vi "GetEventForceActuatorForceWarningField.vi"(10 "Event Data":string, 11 "Cluster in":refnum<vi>) -> (3 "Array":string[](array[string]))   [LabVIEW 2016]
uses:
  SALLV_m1m3/DataTypes/logevent_ForceActuatorForceWarning.ctl
  SALLV_m1m3/SALLV_m1m3.lvlib
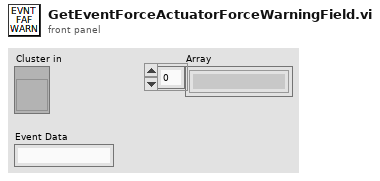
[diagram p1: front panel]
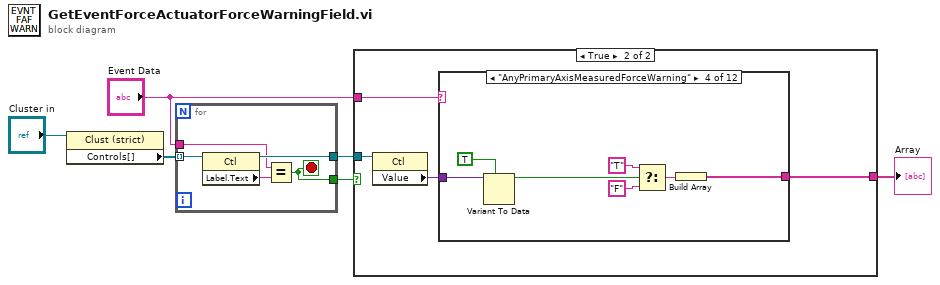
[diagram p0: block diagram]
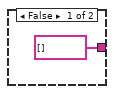
[diagram p2: hidden frame]
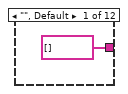
[diagram p3: hidden frame]
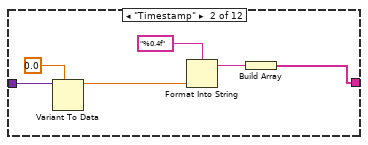
[diagram p4: hidden frame]
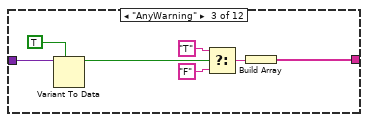
[diagram p5: hidden frame]
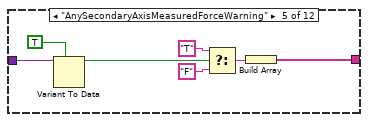
[diagram p6: hidden frame]
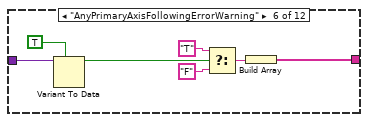
[diagram p7: hidden frame]
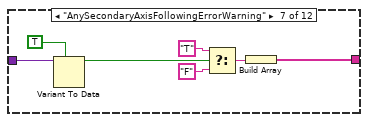
[diagram p8: hidden frame]
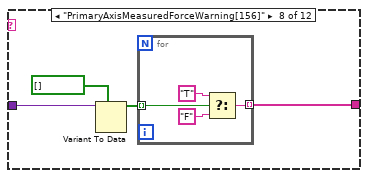
[diagram p9: hidden frame]
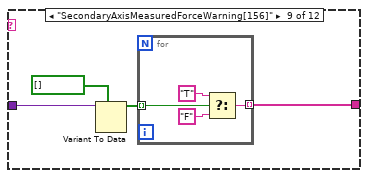
[diagram p10: hidden frame]
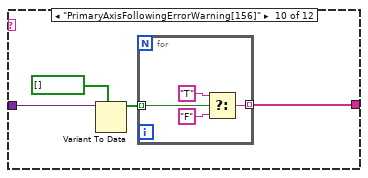
[diagram p11: hidden frame]
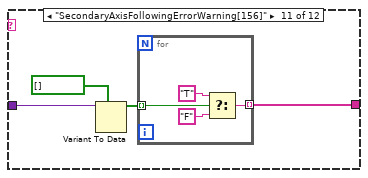
[diagram p12: hidden frame]
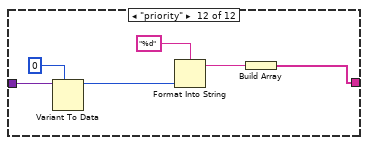
[diagram p13: hidden frame]
diagram:
  n1 = property on="Property Node" class="Clust (strict)"(reference="Cluster in") -> ("Controls[]"=w3:refnum<vi>[])  [unwired: 1 in, 2 out]
  n2 = for {
    tunnel: w3 -> [w11] mode=indexing
    tunnel: [w10] -> w5
    tunnel: "Event Data" -> [w8]
    tunnel: [w7] -> w6
    stop <- w7 stop-if-true
    n3 = property on="Property Node" class="Ctl"(reference=w11) -> (reference out=w10:refnum<vi>, "Label.Text"=w9:string)  [unwired: 1 in, 1 out]
    n4 = Equal?(x=w8, y=w9) -> (x = y?=w7:bool)
  }
  n5 = case shown="True" w6 {
    tunnel: "Event Data" -> [_ w16]
    tunnel: w5 -> [_ w15]
    tunnel: [string[] [] w13] -> w2
    frame False {
    }
    frame True {
      n6 = property on="Property Node" class="Ctl"(reference=w15) -> ("Value"=w14:variant)  [unwired: 1 in, 2 out]
      n7 = case shown="\"AnyPrimaryAxisMeasuredForceWarning\"" w16 {
        tunnel: [string[] [] w21 w24 w31 w38 w45 w52 w59 w67 w75 w83 w94] -> w13
        tunnel: w14 -> [_ w19 w30 w37 w44 w51 w58 w62 w70 w78 w86 w92]
        frame "", Default {
        }
        frame "Timestamp" {
          n8 = Variant To Data(type=0.0, Variant=w19) -> (data=w20:dbl)  [unwired: 1 in, 1 out]
          n9 = Format Into String(format string="%0.4f", w20) -> (resulting string=w22:string)  [unwired: 2 in, 1 out]
          n10 = Build Array(w22) -> (w21:string[])
        }
        frame "AnyWarning" {
          n11 = Variant To Data(type=TRUE, Variant=w30) -> (data=w28:bool)  [unwired: 1 in, 1 out]
          n12 = Select(t="T", s=w28, f="F") -> (s? t:f=w25:string)
          n13 = Build Array(w25) -> (w24:string[])
        }
        frame "AnyPrimaryAxisMeasuredForceWarning" {
          n14 = Variant To Data(type=TRUE, Variant=w37) -> (data=w35:bool)  [unwired: 1 in, 1 out]
          n15 = Select(t="T", s=w35, f="F") -> (s? t:f=w32:string)
          n16 = Build Array(w32) -> (w31:string[])
        }
        frame "AnySecondaryAxisMeasuredForceWarning" {
          n17 = Variant To Data(type=TRUE, Variant=w44) -> (data=w42:bool)  [unwired: 1 in, 1 out]
          n18 = Select(t="T", s=w42, f="F") -> (s? t:f=w39:string)
          n19 = Build Array(w39) -> (w38:string[])
        }
        frame "AnyPrimaryAxisFollowingErrorWarning" {
          n20 = Variant To Data(type=TRUE, Variant=w51) -> (data=w49:bool)  [unwired: 1 in, 1 out]
          n21 = Select(t="T", s=w49, f="F") -> (s? t:f=w46:string)
          n22 = Build Array(w46) -> (w45:string[])
        }
        frame "AnySecondaryAxisFollowingErrorWarning" {
          n23 = Variant To Data(type=TRUE, Variant=w58) -> (data=w56:bool)  [unwired: 1 in, 1 out]
          n24 = Select(t="T", s=w56, f="F") -> (s? t:f=w53:string)
          n25 = Build Array(w53) -> (w52:string[])
        }
        frame "PrimaryAxisMeasuredForceWarning[156]" {
          n26 = Variant To Data(type=bool[] [], Variant=w62) -> (data=w60:bool[])  [unwired: 1 in, 1 out]
          n27 = for {
            tunnel: w60 -> [w66] mode=indexing
            tunnel: [w63] -> w59 mode=indexing
            n28 = Select(t="T", s=w66, f="F") -> (s? t:f=w63:string)
          }
        }
        frame "SecondaryAxisMeasuredForceWarning[156]" {
          n29 = Variant To Data(type=bool[] [], Variant=w70) -> (data=w68:bool[])  [unwired: 1 in, 1 out]
          n30 = for {
            tunnel: w68 -> [w74] mode=indexing
            tunnel: [w71] -> w67 mode=indexing
            n31 = Select(t="T", s=w74, f="F") -> (s? t:f=w71:string)
          }
        }
        frame "PrimaryAxisFollowingErrorWarning[156]" {
          n32 = Variant To Data(type=bool[] [], Variant=w78) -> (data=w76:bool[])  [unwired: 1 in, 1 out]
          n33 = for {
            tunnel: w76 -> [w82] mode=indexing
            tunnel: [w79] -> w75 mode=indexing
            n34 = Select(t="T", s=w82, f="F") -> (s? t:f=w79:string)
          }
        }
        frame "SecondaryAxisFollowingErrorWarning[156]" {
          n35 = Variant To Data(type=bool[] [], Variant=w86) -> (data=w84:bool[])  [unwired: 1 in, 1 out]
          n36 = for {
            tunnel: w84 -> [w90] mode=indexing
            tunnel: [w87] -> w83 mode=indexing
            n37 = Select(t="T", s=w90, f="F") -> (s? t:f=w87:string)
          }
        }
        frame "priority" {
          n38 = Variant To Data(type=0, Variant=w92) -> (data=w93:i32)  [unwired: 1 in, 1 out]
          n39 = Format Into String(format string="%d", w93) -> (resulting string=w95:string)  [unwired: 2 in, 1 out]
          n40 = Build Array(w95) -> (w94:string[])
        }
      }
    }
  }
  "Array" <- w2
